vi "Settings_init.vi"(2 "error in":errorcluster) -> (0 "error out":errorcluster)   [LabVIEW 2009, in "Utility.lvlib"]
uses:
  Utility.lvlib
  <vilib>/Utility/config.llb/Read Key (String).vi
  <vilib>/Utility/config.llb/NI_LVConfig.lvlib
panel:
  out "appended path":path
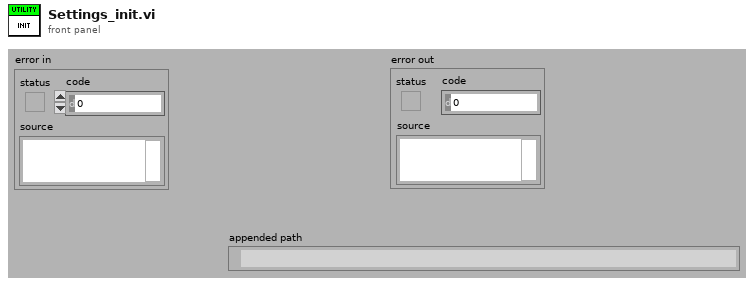
[diagram p1: front panel]
types:
  T1 = typedef "NI_LVConfig.lvlib/Config Data RefNum.ctl" = refnum<k1>
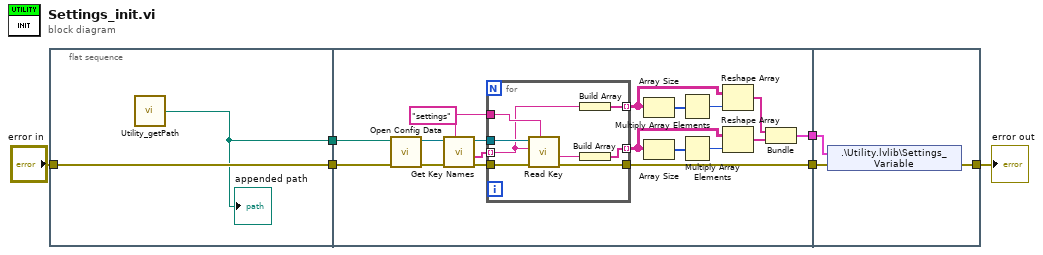
[diagram p0: block diagram]
diagram:
  n1 = flat-sequence {
    tunnel: [w7] -> w6
    tunnel: "error in" -> [w8]
    tunnel: [w8] -> w4
    tunnel: w6 -> [w26]
    tunnel: w4 -> [w25]
    tunnel: [w19] -> w3
    tunnel: [w9] -> w2
    tunnel: w3 -> [w36]
    tunnel: w2 -> [w37]
    tunnel: [w35] -> w1
    frame #0 {
      n2 = call "Utility_getPath.vi"() -> ("appended path"=w7:path)  [unwired: 5 in]
      "appended path" <- w7
    }
    frame #1 {
      w20 = "settings" ("section")
      n3 = call <vilib>:"Open Config Data.vi"("error in (no error)"=w25, "configuration file path"=w26) -> ("error out"=w24:errorcluster, "refnum"=w23:T1)  [unwired: 7 in, 1 out]
      n4 = call <vilib>:"Get Key Names.vi"("section"=w20, "error in (no error)"=w24, "refnum"=w23) -> ("error out"=w22:errorcluster, "key names"=w18:string[], "refnum out"=w21:T1)  [unwired: 5 in, 1 out]
      n5 = for {
        tunnel: w22 -> [w34]
        tunnel: w18 -> [w28] mode=indexing
        tunnel: w21 -> [w33]
        tunnel: w20 -> [w32]
        tunnel: [w30] -> w11 mode=indexing
        tunnel: [w29] -> w19
        tunnel: [w27] -> w15 mode=indexing
        n6 = call-poly <vilib>:"Read Key.vi"("section"=w32, "error in (no error)"=w34, "key"=w28, "refnum"=w33) -> ("error out"=w29:errorcluster, "value"=w31:string)  [unwired: 4 in, 2 out]
        n7 = Build Array(w28) -> (w27:string[])
        n8 = Build Array(w31) -> (w30:string[])
      }
      n9 = Array Size(array=w15) -> (size(s)=w17:i32[])
      n10 = Array Size(array=w11) -> (size(s)=w13:i32[])
      n11 = Multiply Array Elements(1:w17) -> (0:w16:i32)
      n12 = Multiply Array Elements(1:w13) -> (0:w12:i32)
      n13 = Reshape Array(w15, w16) -> (w14:string[])
      n14 = Reshape Array(w11, w12) -> (w10:string[])
      n15 = Bundle(w14, w10) -> (w9:cluster{string[], string[]})  [unwired: 1 in]
    }
    frame #2 {
      n16 = shared-variable ".\\Utility.lvlib\\Settings_Variable"(w37, error in=w36) -> (error out=w35:errorcluster)
    }
  }
  "error out" <- w1
